vi "Request Data Persistence.vi"(4 "Initialize Persistence If None Found? (T)":bool=TRUE, 6 "One Shot? (F)":bool, 7 "Persistence Folder Path":path, 8 "error in (no error)":errorcluster, 9 "Data Type/Initial Value":variant, 10 "Datum Name":string, 11 "IObserver in":refnum<class "IObserver.lvclass">) -> (0 "error out":errorcluster, 2 "Subscription Policy":T1, 3 "IObserver out":refnum<class "IObserver.lvclass">)   [LabVIEW 2020, in "IObserver.lvlib" / "IObserver.lvclass"]
doc: "<License>\nCopyright © 2017 Composed Systems, LLC | All rights reserved\nwww.composed.io\n\nAuthor: Ethan Stern <ethan.stern@composed.io>\n\nThis software is provided \"AS IS\" WITHOUT WARRANTIES, either express or implied, AND IS FOR EDUCATIONAL PURPOSES ONLY.\n</License>"
uses:
  <vilib>/gpm_packages/@cs/mva-core/Source/IObserver/IObserver/IObserver.lvclass
  C:/Program Files/National Instruments/LabVIEW 2020/vi.lib/ActorFramework/Actor/Actor.lvclass
  <vilib>/gpm_packages/@cs/mva-core/Source/IMediator/ISubscriptionPolicy/ISubscriptionPolicy Reference.ctl
  <vilib>/gpm_packages/@cs/mva-core/Source/IMediator/ISubscriptionPolicy/ISubscriptionPolicy.lvclass
  <vilib>/ActorFramework/Actor/Actor.lvclass/Actor.ctl
  <vilib>/ActorFramework/Message Enqueuer/Message Enqueuer.lvclass/Message Enqueuer.ctl
  <vilib>/gpm_packages/@cs/mva-core/Source/SubscriptionPolicy/ValueChangeSubscription/ValueChangeSubscription.lvclass/ValueChangeSubscription.ctl
  <vilib>/gpm_packages/@cs/mva-core/Source/SubscriptionPolicy/OneShotSubscription/OneShotSubscription.lvclass/OneShotSubscription.ctl
  <vilib>/gpm_packages/@cs/transport/Source/Concrete/PersistToDiskTransport/PersistToDiskTransport.lvclass/PersistToDiskTransport.ctl
  <vilib>/gpm_packages/@cs/mva-core/Source/IMediator/SubscriptionRequest/SubscriptionRequest.lvclass/SubscriptionRequest.ctl
  <vilib>/gpm_packages/@cs/mva-core/Source/IObserver/IObserver Messages/Subscribe Msg/Subscribe Msg.lvclass/Subscribe Msg.ctl
  <vilib>/ActorFramework/Message Enqueuer/Init from Existing Queue.vi
  <vilib>/ActorFramework/Message Enqueuer/Enqueue.vi
  <vilib>/gpm_packages/@cs/transport/Source/Concrete/PersistToDiskTransport/Format Persistent Filename.vi
  <vilib>/Utility/error.llb/Clear Errors.vi
  <vilib>/gpm_packages/@cs/mva-core/Source/SubscriptionPolicy/ValueChangeSubscription/ValueChangeSubscription.lvclass
  C:/Program Files/National Instruments/LabVIEW 2020/vi.lib/gpm_packages/@cs/mva-core/Source/IMediator/ISubscriptionPolicy/ISubscriptionPolicy.lvclass
  <vilib>/gpm_packages/@cs/mva-core/Source/SubscriptionPolicy/OneShotSubscription/OneShotSubscription.lvclass
  <vilib>/gpm_packages/@cs/transport/Source/Concrete/PersistToDiskTransport/PersistToDiskTransport.lvclass
  C:/Program Files/National Instruments/LabVIEW 2020/vi.lib/gpm_packages/@cs/transport/Source/ITransport/ITransport.lvclass
  <vilib>/gpm_packages/@cs/mva-core/Source/IObserver/IObserver Messages/Subscribe Msg/Subscribe Msg.lvclass
  C:/Program Files/National Instruments/LabVIEW 2020/vi.lib/ActorFramework/Message/Message.lvclass
  <vilib>/gpm_packages/@cs/variant/Source/Format Type String.vi
  <vilib>/Utility/error.llb/Error Cluster From Error Code.vi
  <vilib>/ActorFramework/Message Priority Queue/Priority Enqueue.vi
  <vilib>/gpm_packages/@cs/mva-core/Source/IMediator/SubscriptionRequest/SubscriptionRequest.lvclass
  <vilib>/ActorFramework/Message Enqueuer/Message Enqueuer.lvclass
  <vilib>/gpm_packages/@cs/transport/Source/ITransport/ITransport.lvclass
  <vilib>/ActorFramework/Actor/Actor.lvclass
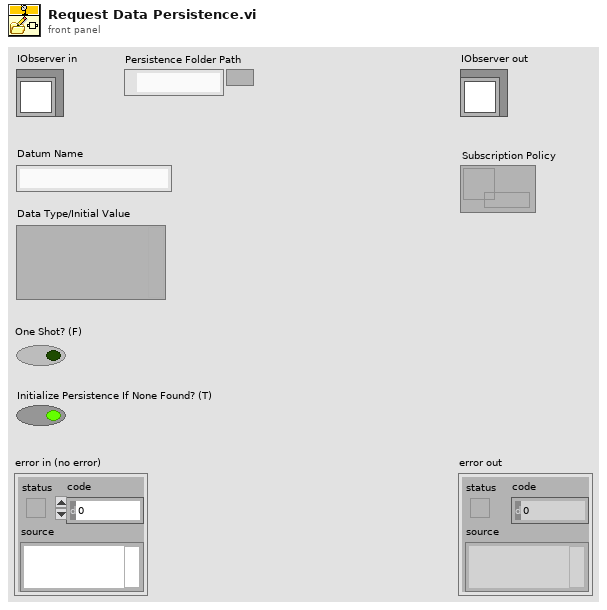
[diagram p1: front panel]
types:
  T1 = typedef "IMediator.lvlib/ISubscriptionPolicy.lvclass/ISubscriptionPolicy Reference.ctl" = refnum<data-value>
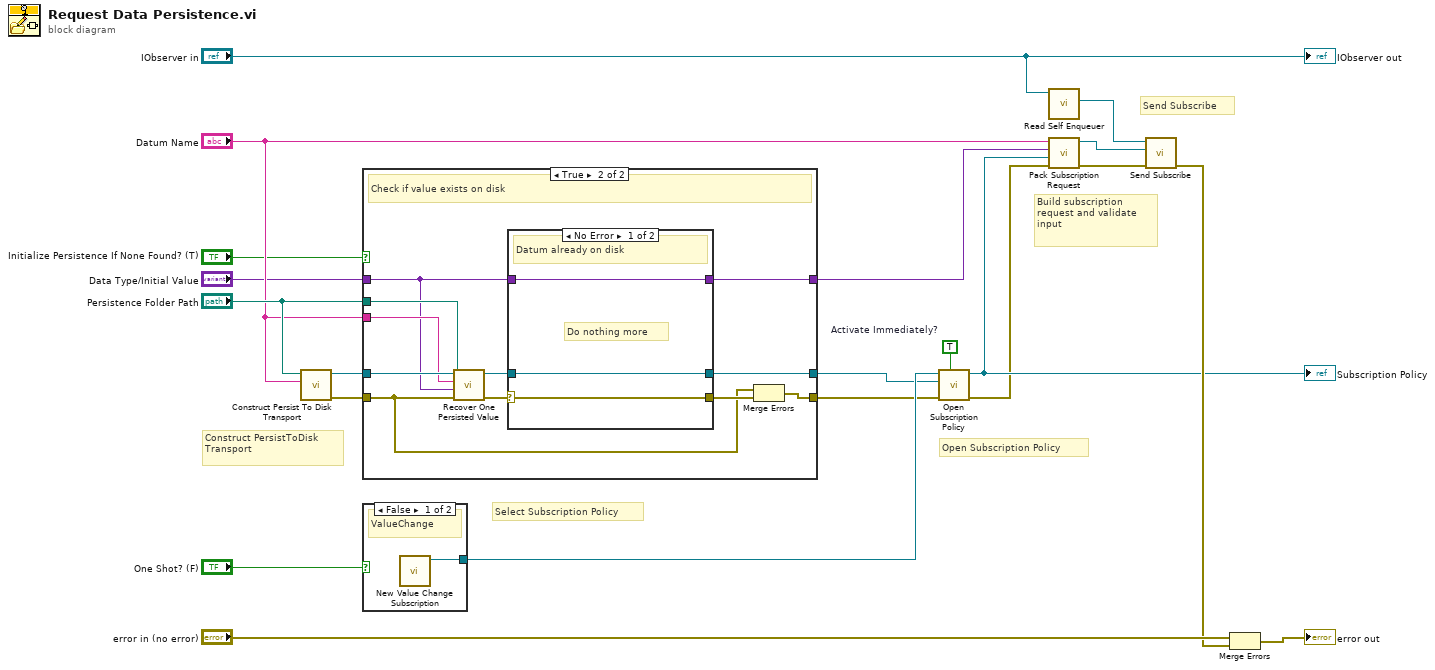
[diagram p0: block diagram]
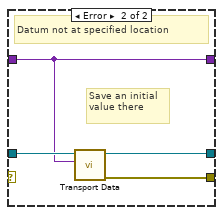
[diagram p3: hidden frame]
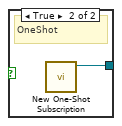
[diagram p4: hidden frame]
diagram:
  w14 = TRUE  # Activate Immediately?
  # "Open Subscription Policy"
  # "Select Subscription Policy"
  # "Send Subscribe"
  # "Build subscription\nrequest and validate\ninput"
  # "Construct PersistToDisk\nTransport"
  n1 = call <vilib>:"Construct Persist To Disk Transport.vi"("Datum Name"="Datum Name", "Folder Path"="Persistence Folder Path") -> ("error out"=w8:errorcluster, "PersistToDiskTransport"=w4:refnum<class "PersistToDiskTransport.lvclass">)  [unwired: 8 in]
  n2 = case shown="True" "Initialize Persistence If None Found? (T)" {
    tunnel: "Persistence Folder Path" -> [_ w34]
    tunnel: "Datum Name" -> [_ w26]
    tunnel: "Data Type/Initial Value" -> [w24 w25]
    tunnel: w8 -> [w23 w27]
    tunnel: [w23 w28] -> w5
    tunnel: [w24 w29] -> w7
    tunnel: w4 -> [w22 w31]
    tunnel: [w22 w30] -> w3
    frame False {
      # "Subscribing only"
    }
    frame True {
      # "Check if value exists on disk"
      n3 = call <vilib>:"Recover One Persisted Value.vi"("error in (no error)"=w27, "Data Type"=w25, "Datum Name"=w26, "Folder Path"=w34) -> ("error out"=w33:errorcluster)  [unwired: 6 in, 1 out]
      n4 = case shown="No Error" w33 {
        selector: w33 -> [w35 _]
        tunnel: [w35 w41] -> w32
        tunnel: w31 -> [w36 w40]
        tunnel: [w36 w39] -> w30
        tunnel: w25 -> [w37 w38]
        tunnel: [w37 w38] -> w29
        frame No Error {
          # "Do nothing more"
          # "Datum already on disk"
        }
        frame Error {
          # "Save an initial\nvalue there"
          # "Datum not at specified location"
          n5 = call <vilib>:"Transport Data.vi"("Value"=w38, "ITransport in"=w40) -> ("error out"=w41:errorcluster, "ITransport out"=w39:refnum<class "PersistToDiskTransport.lvclass">)  [unwired: 8 in]
        }
      }
      n6 = Merge Errors(w27, w32) -> (w28:errorcluster)
    }
  }
  n7 = case shown="False" "One Shot? (F)" {
    tunnel: [w42 w43] -> w12
    frame False {
      # "ValueChange"
      n8 = call <vilib>:"New Value Change Subscription.vi"() -> ("ValueChangeSubscription Out"=w42:refnum<class "ValueChangeSubscription.lvclass">)  [unwired: 11 in]
    }
    frame True {
      # "OneShot"
      n9 = call <vilib>:"New One-Shot Subscription.vi"() -> ("OneShotSubscription Out"=w43:refnum<class "OneShotSubscription.lvclass">)  [unwired: 11 in]
    }
  }
  n10 = call <vilib>:"Open Subscription Policy.vi"("Activate? (T)"=w14, "error in (no error)"=w5, "Transport"=w3, "SubscriptionPolicy"=w12) -> ("error out"=w2:errorcluster, "Subscription Policy"=w13:T1)  [unwired: 6 in]
  "Subscription Policy" <- w13
  n11 = call <vilib>:"Read Self Enqueuer.vi"("Actor"="IObserver in") -> ("Self Enqueuer"=w15:refnum<class "Message Enqueuer.lvclass">)  [unwired: 10 in]
  n12 = call <vilib>:"Pack Subscription Request.vi"("error in (no error)"=w2, "Subscription Policy"=w13, "Type"=w7, "Datum Name"="Datum Name") -> ("error out"=w1:errorcluster, "SubscriptionRequest"=w17:refnum<class "SubscriptionRequest.lvclass">)  [unwired: 6 in]
  n13 = call <vilib>:"Send Subscribe.vi"("error in (no error)"=w1, "SubscriptionRequest"=w17, "Message Enqueuer"=w15) -> ("error out"=w16:errorcluster)  [unwired: 7 in, 1 out]
  n14 = Merge Errors("error in (no error)", w16) -> (→"error out":errorcluster)
  "IObserver out" <- "IObserver in"
